vi "updateTime.vi"(8 "error in (no error)":errorcluster, 10 "time":dbl, 11 "ScriptEvent in":refnum<class "ScriptEvent.lvclass">) -> (0 "error out":errorcluster, 2 "dt":dbl, 3 "ScriptEvent out":refnum<class "ScriptEvent.lvclass">)   [LabVIEW 2011, in "Tools.lvlib" / "Scripting.lvlib" / "ScriptEvent.lvclass"]
uses:
  ScriptEvent.lvclass
  ScriptEvent.lvclass/ScriptEvent.ctl
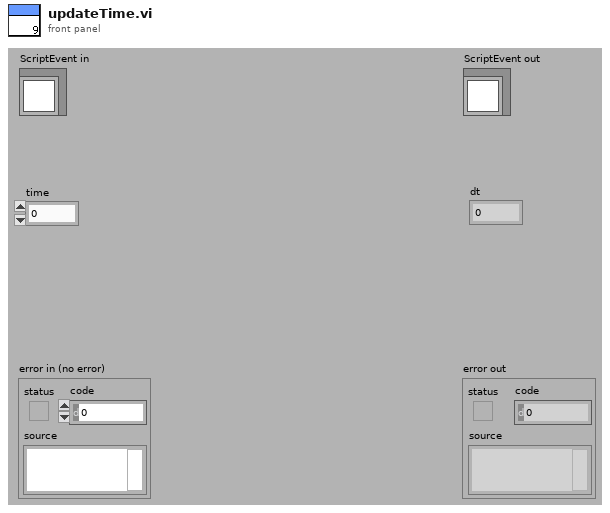
[diagram p1: front panel]
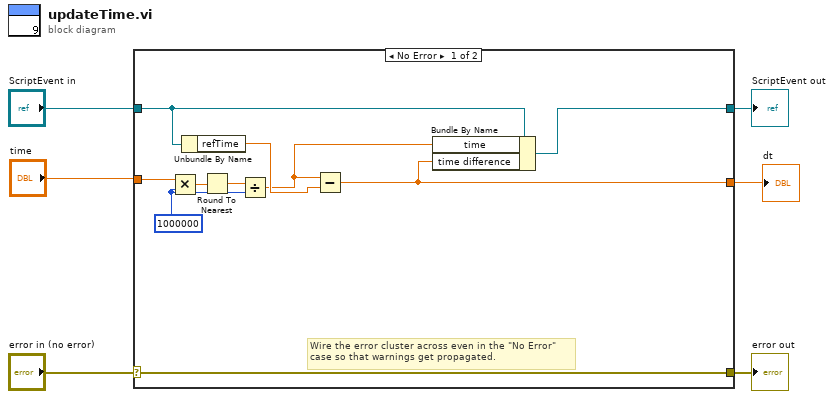
[diagram p0: block diagram]
diagram:
  n1 = case shown="No Error" "error in (no error)" {
    selector: "error in (no error)" -> [w16 w18]
    tunnel: [w16 w18] -> w5
    tunnel: [w12 w17] -> w3
    tunnel: "ScriptEvent in" -> [w13 w17]
    tunnel: "time" -> [w11 _]
    tunnel: [w14 _] -> w1
    frame No Error {
      w8 = 1000000
      # "Wire the error cluster across even in the \"No Error\"\ncase so that warnings get propagated."
      n2 = Multiply(x=w11, y=w8) -> (x*y=w10:dbl)
      n3 = Unbundle By Name(w13) -> ("refTime"=w15:dbl)
      n4 = Round To Nearest(number=w10) -> (nearest integer value=w9:dbl)
      n5 = Divide(x=w9, y=w8) -> (x/y=w7:dbl)
      n6 = Subtract(x=w7, y=w15) -> (x-y=w14:dbl)
      n7 = Bundle By Name(cluster=w13, "time"=w7, "time difference"=w14) -> (w12:refnum<class "ScriptEvent.lvclass">)
    }
    frame Error {
    }
  }
  "error out" <- w5
  "ScriptEvent out" <- w3
  "dt" <- w1
